vi "GSI-HVSwitch2.destructor.vi"(0 "i ref in":refnum<vi>, 5 "error in (no error)":errorcluster) -> (19 "error out":errorcluster)   [LabVIEW 2014, in "GSI-HVSwitch2.lvlib"]
doc: "This is the destructor of a class.\n\nLicense Agreement for this software:\n\nCopyright (C)\nGesellschaft für Schwerionenforschung, GSI\nPlanckstr. 1\n64291 Darmstadt\nGermany\n\nContact: D.Beck@gsi.de \n\nThis program is free software; you can redistribute it and/or modify it under the terms of the \nGNU General Public License as published by the Free Software Foundation; either version 2 of \nthe license, or (at your option) any later version.\n\nThis program is distributed in the hope that it will be useful, but WITHOUT ANY WARRANTY; \nwithout even the implied warranty of MERCHANTABILITY or FITNESS FOR A PARTICULAR PURPOSE. See the GNU General License for more details (http://www.gnu.org).\n\nGesellschaft für Schwerionenforschung, GSI\nPlanckstr. 1, 64291 Darmstadt, Germany\nFor all questions and ideas contact: M.Richter@gsi.de, H.Brand@gsi.de or D.Beck@gsi.de.\nLast update: 16-JUN-2004"
uses:
  GSI-HVSwitch2.lvlib
  CSlibraries-extern/DimLVEvent/LVDimInterface/LVDimInterface.lvlib
  CSCore/CSApplicationBaseClasses/PSChannelBase/PSChannelBase.lvlib
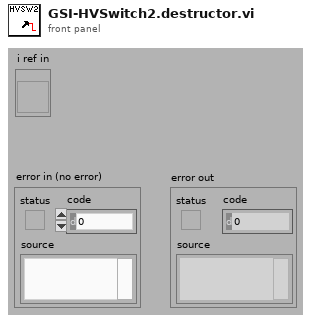
[diagram p1: front panel]
types:
  T1 = typedef "GSI-HVSwitch2.lvlib/GSI-HVSwitch2.i attribute.ctl" = cluster{"SDEX VISA Cluster":T2, "SetVoltage SW0":dbl, "SetVoltage SW1":dbl, "ActTempAmp":dbl, "ActTempPS1":dbl, "ActTempPS2":dbl, "mode":T5, "interfaceInitialized":bool, "serviceIDs":cluster{"nomVoltage0ID":i32, "nomVoltage1ID":i32, "actTempAmpID":i32, "actTempPS1ID":i32, "actTempPS2ID":i32, "modeID":i32}, "usedChannels":i32}
  T2 = typedef "SDEXDriver.lvlib/SDEX.VISA Control.ctl" = cluster{"VISA resource name":refnum<visa-resource-name>, "HEX address":u16, "VISA Timeout Value (1000 ms)":u32, "Lock Timeout (1000 ms)":u32, "semaphore":T3, "Baud rate":u32, "revision":T4, "deviceInfo":string}
  T3 = typedef "Semaphore RefNum" = refnum<k1>
  T4 = typedef "SDEXDriver.lvlib/SDEX.revisionType.ctl" = enum16{"unknown", "hvamp3", "hvswi1", "htrp0", "WDG0"}
  T5 = typedef "GSI-HVSwitch2.lvlib/GSI-HVSwitch2.mode.ctl" = enum16{"unknown", "switch", "stepper"}
  T6 = enum16{"SetAttribute", "GetAttribute", "CreateAttribute", "DestroyAttribute", "DestroyAllAtributes"}
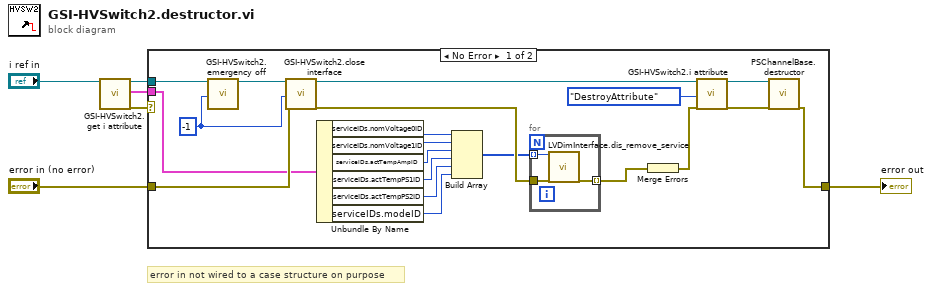
[diagram p0: block diagram]
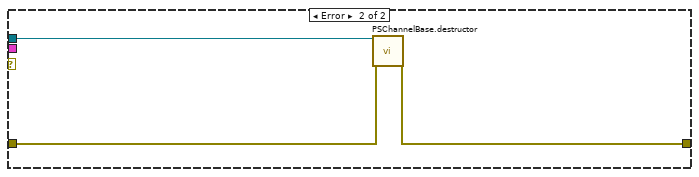
[diagram p2: hidden frame]
diagram:
  # "error in not wired to a case structure on purpose"
  n1 = call "GSI-HVSwitch2.get i attribute.vi"("i ref in"="i ref in") -> ("i ref out"=w3:refnum<vi>, "i attribute"=w1:T1, "error out"=w2:errorcluster)  [unwired: 16 in]
  n2 = case shown="No Error" w2 {
    tunnel: [w23 w30] -> w6
    tunnel: "error in (no error)" -> [w22 w31]
    tunnel: w3 -> [w17 w32]
    tunnel: w1 -> [w20 _]
    frame No Error {
      w15 = -1 ("ms timeout (10000)")
      n3 = call "GSI-HVSwitch2.emergency off.vi"("i ref in"=w17, "ms timeout (10000)"=w15) -> ("i ref out"=w16:refnum<vi>)  [unwired: 15 in, 2 out]
      n4 = call "GSI-HVSwitch2.close interface.vi"("i ref in"=w16, "ms timeout (10000)"=w15, "error in (no error)"=w22) -> ("i ref out"=w21:refnum<vi>, "error out"=w19:errorcluster)  [unwired: 14 in, 1 out]
      n5 = Unbundle By Name(w20) -> ("serviceIDs.nomVoltage0ID"=w14:i32, "serviceIDs.nomVoltage1ID"=w13:i32, "serviceIDs.actTempAmpID"=w12:i32, "serviceIDs.actTempPS1ID"=w11:i32, "serviceIDs.actTempPS2ID"=w10:i32, "serviceIDs.modeID"=w9:i32)
      n6 = Build Array(w14, w13, w12, w11, w10, w9) -> (w8:i32[])
      n7 = for {
        tunnel: w19 -> [w29]
        tunnel: w8 -> [w28] mode=indexing
        tunnel: [w27] -> w7 mode=indexing
        n8 = call "LVDimInterface.dis_remove_service.vi"("my_serviceID"=w28, "error in (no error)"=w29) -> ("error out"=w27:errorcluster)  [unwired: 17 in]
      }
      n9 = Merge Errors(w7) -> (w18:errorcluster)
      n10 = call "GSI-HVSwitch2.i attribute.vi"("VI Refnum"=w21, "Action"=T6."DestroyAttribute", "error in (no error)"=w18) -> ("VI Refnum out"=w25:refnum<vi>, "error out"=w24:errorcluster)  [unwired: 14 in, 1 out]
      n11 = call "PSChannelBase.destructor.vi"("i ref in"=w25, "error in (no error)"=w24) -> ("error out"=w23:errorcluster)  [unwired: 17 in]
    }
    frame Error {
      n12 = call "PSChannelBase.destructor.vi"("i ref in"=w32, "error in (no error)"=w31) -> ("error out"=w30:errorcluster)  [unwired: 17 in]
    }
  }
  "error out" <- w6
